vi "Relógio despertador.vi"() -> ()   [LabVIEW 2018]
panel:
  out "Boolean":bool
  out "Display Alarme":dbl format="%<%H:%M:%S>T"
  in  "Minutos":bool
  in  "Horas":bool
  in  "stop":bool
  in  "Alarm":bool
  in  "Alarme SET":bool
  out "Display Horas":dbl format="%<%H:%M:%S>T"
  # "OFF / ON"
  # "OFF / ON"
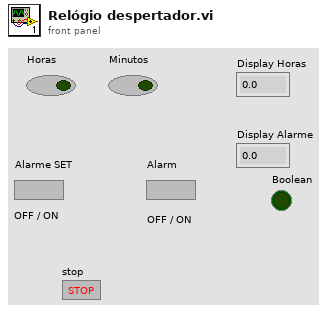
[diagram p1: front panel]
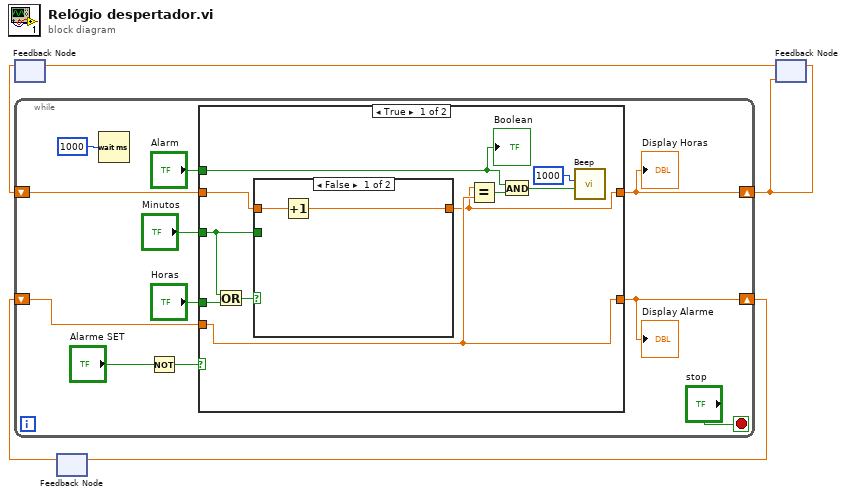
[diagram p0: block diagram]
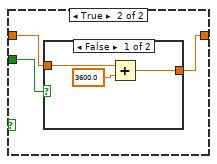
[diagram p2: hidden frame]
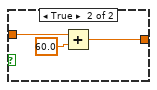
[diagram p3: hidden frame]
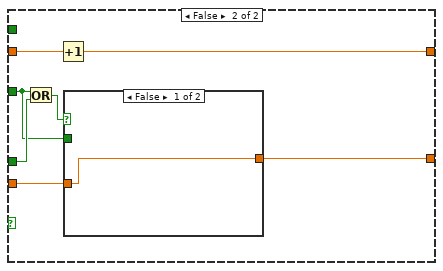
[diagram p4: hidden frame]
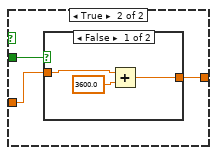
[diagram p5: hidden frame]
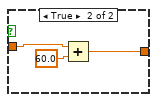
[diagram p6: hidden frame]
diagram:
  n1 = feedback #1() -> (w4:dbl)  [unwired: 1 in]
  n2 = feedback #2() -> (w1:dbl)  [unwired: 1 in]
  n3 = while {
    shift-right: [w13] -> w3
    shift-left: w4 -> [w11]
    shift-right: [w8] -> w2
    shift-left: w1 -> [w7]
    stop <- "stop" stop-if-true
    n4 = Wait (ms)(milliseconds to wait=u32 1000 ("millisecond multiple")) -> ()  [unwired: 1 out]
    n5 = Not(x="Alarme SET") -> (.not. x?=w9:bool)
    n6 = case shown="True" w9 {
      tunnel: "Horas" -> [w26 w44]
      tunnel: [w20 w38] -> w13
      tunnel: "Minutos" -> [w24 w42]
      tunnel: w11 -> [w23 w39]
      tunnel: [w21 w41] -> w8
      tunnel: w7 -> [w21 w40]
      tunnel: "Alarm" -> [w17 _]
      frame True {
        n7 = Or(x=w24, y=w26) -> (x .or. y?=w25:bool)
        n8 = case shown="False" w25 {
          tunnel: [w28 w30] -> w20
          tunnel: w24 -> [_ w31]
          tunnel: w23 -> [w27 w29]
          frame False {
            n9 = Increment(x=w27) -> (x+1=w28:dbl)
          }
          frame True {
            n10 = case shown="False" w31 {
              tunnel: [w33 w36] -> w30
              tunnel: w29 -> [w32 w35]
              frame False {
                n11 = Add(x=w32, y=3600.0) -> (x+y=w33:dbl)
              }
              frame True {
                n12 = Add(x=w35, y=60.0) -> (x+y=w36:dbl)
              }
            }
          }
        }
        n13 = Equal?(x=w20, y=w21) -> (x = y?=w22:bool)
        n14 = And(x=w17, y=w22) -> (x .and. y?=w18:bool)
        n15 = call <vilib>:"Beep.vi"("use system alert? (T)"=w18, "duration (msec)"=u32 1000) -> ()  [unwired: 10 in]
        "Boolean" <- w17
      }
      frame False {
        n16 = Or(x=w42, y=w44) -> (x .or. y?=w43:bool)
        n17 = Increment(x=w39) -> (x+1=w38:dbl)
        n18 = case shown="False" w43 {
          tunnel: [w45 w47] -> w41
          tunnel: w42 -> [_ w48]
          tunnel: w40 -> [w45 w46]
          frame False {
          }
          frame True {
            n19 = case shown="False" w48 {
              tunnel: [w50 w53] -> w47
              tunnel: w46 -> [w49 w52]
              frame False {
                n20 = Add(x=w49, y=3600.0) -> (x+y=w50:dbl)
              }
              frame True {
                n21 = Add(x=w52, y=60.0) -> (x+y=w53:dbl)
              }
            }
          }
        }
      }
    }
    "Display Horas" <- w13
    "Display Alarme" <- w8
  }
  n22 = feedback-in #2(w2) -> ()
  n23 = feedback-in #3(w3) -> ()
  n24 = feedback #3(w3) -> (w5:dbl)
  n25 = feedback-in #1(w5) -> ()
